vi "Image_Crop.vi"(6 "Shrink":bool, 7 "ROI Descriptor":T2 {"Contours"."Type" items=["No Selection", "Point", "Line", "Rectangle", "Oval", "Polygon", "Free", "Annulus", "Unused2", "Unused3", "Broken Line", "Free Hand Line", "Rotated Rectangle"]}, 8 "error in (no error)":errorcluster, 9 "Out / In":bool, 10 "Image Dest":T1, 11 "Image Src":T1) -> (0 "error out":errorcluster, 3 "Image Out":T1)   [LabVIEW 2022 SP3]
uses:
  <vilib>/vision/Image Controls.llb/IMAQ Image.ctl
  <vilib>/vision/NI_Vision_Development_Module.lvlib
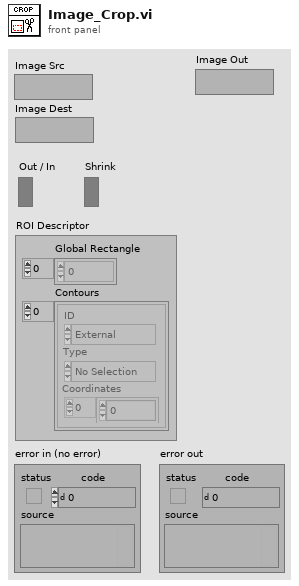
[diagram p1: front panel]
types:
  T1 = typedef "IMAQ Image.ctl" = refnum<image>
  T2 = cluster{"Global Rectangle":i32[], "Contours":cluster{"ID":enum32{"External", "Internal"}, "Type":u32, "Coordinates":i32[]}[]}
  T3 = cluster{"ID":enum32{"External", "Internal"}, "Type":u32, "Coordinates":i32[]}[]
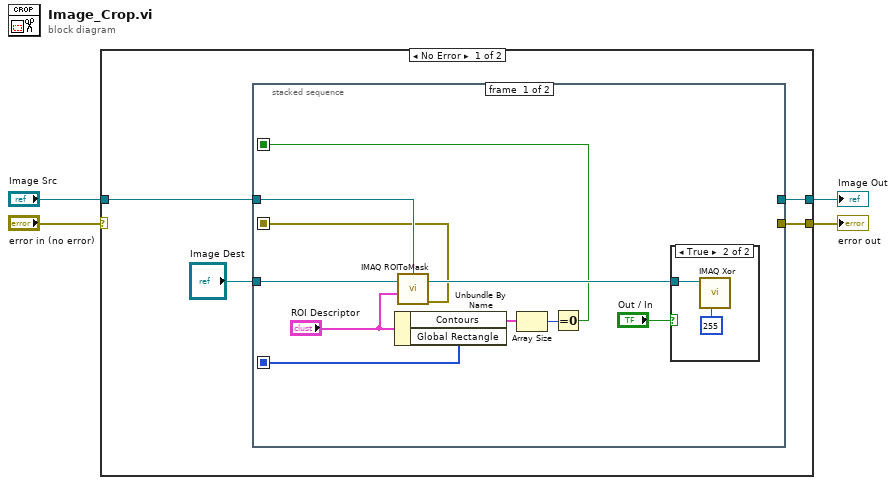
[diagram p0: block diagram]
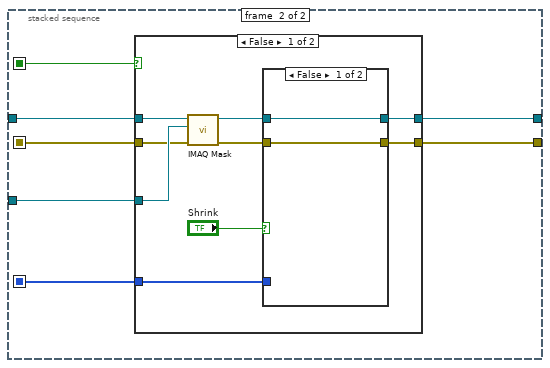
[diagram p3: hidden frame]
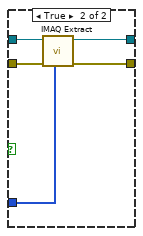
[diagram p4: hidden frame]
diagram:
  n1 = case shown="No Error" "error in (no error)" {
    selector: "error in (no error)" -> [_ w47]
    tunnel: [w8 w47] -> w4
    tunnel: "Image Src" -> [w7 w46]
    tunnel: [w6 w46] -> w2
    frame No Error {
      n2 = stacked-sequence {
        seq-local: [w10 _] -> [_ w27]
        seq-local: [w15 _] -> [_ w24]
        seq-local: [w9 _] -> [_ w22]
        tunnel: w7 -> [w16 w26]
        tunnel: "Image Dest" -> [w18 w25]
        tunnel: [_ w21] -> w8
        tunnel: [_ w23] -> w6
        frame #0 {
          n3 = Unbundle By Name("ROI Descriptor") -> ("Contours"=w11:T3, "Global Rectangle"=w10:i32[])
          n4 = call "IMAQ ROIToMask"("ROI Descriptor"="ROI Descriptor", "Image"=w18, "Image Model"=w16) -> ("error out"=w9:errorcluster, "Image Out"=w17:T1)  [unwired: 2 in, 2 out]
          n5 = Array Size(array=w11) -> (size(s)=w14:i32)
          n6 = Equal To 0?(x=w14) -> (x = 0?=w15:bool)
          n7 = case shown="True" "Out / In" {
            tunnel: w17 -> [_ w20]
            frame False {
            }
            frame True {
              n8 = call "IMAQ Xor"("Constant"=255, "Image Src A"=w20) -> ()  [unwired: 4 in, 6 out]
            }
          }
        }
        frame #1 {
          n9 = case shown="False" w24 {
            tunnel: w27 -> [w36 _]
            tunnel: [w35 w45] -> w23
            tunnel: w26 -> [w34 w45]
            tunnel: w25 -> [w32 _]
            tunnel: w22 -> [w30 w44]
            tunnel: [w28 w44] -> w21
            frame False {
              n10 = call "IMAQ Mask"("error in (no error)"=w30, "Image Mask"=w32, "Image Src"=w34) -> ("error out"=w29:errorcluster, "Image Dst Out"=w33:T1)  [unwired: 1 in, 1 out]
              n11 = case shown="False" "Shrink" {
                tunnel: w33 -> [w38 w43]
                tunnel: w36 -> [_ w42]
                tunnel: [w38 w41] -> w35
                tunnel: w29 -> [w37 w40]
                tunnel: [w37 w39] -> w28
                frame False {
                }
                frame True {
                  n12 = call "IMAQ Extract"("Optional Rectangle"=w42, "error in (no error)"=w40, "Image Src"=w43) -> ("error out"=w39:errorcluster, "Image Dst Out"=w41:T1)  [unwired: 3 in, 4 out]
                }
              }
            }
            frame True {
            }
          }
        }
      }
    }
    frame Error {
    }
  }
  "error out" <- w4
  "Image Out" <- w2
